vi "Autotest_Instr.vi"(8 "error in (no error)":errorcluster caption="entrée d'erreur (pas d'erreur)", 11 "Class Instrument (Default) en entrée":refnum<class "Class Instrument (Default).lvclass">) -> (0 "error out":errorcluster caption="sortie d'erreur", 3 "Class Instrument (Default) en sortie":refnum<class "Class Instrument (Default).lvclass">)   [LabVIEW 2020, in "Library Instrument & Equipement.lvlib" / "Library Instruments.lvlib" / "Class Instrument (Default).lvclass"]
uses:
  Class Instrument (Default).lvclass
  Class Instrument (Default).lvclass/Class Instrument (Default).ctl
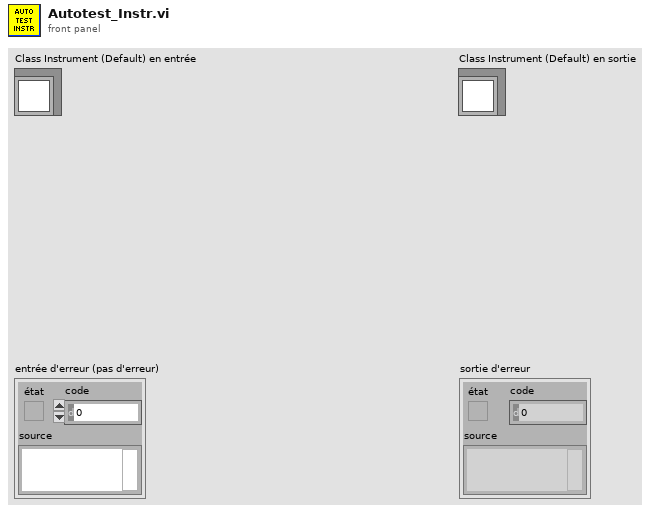
[diagram p1: front panel]
types:
  T1 = typedef "Semaphore RefNum" = refnum<k1>
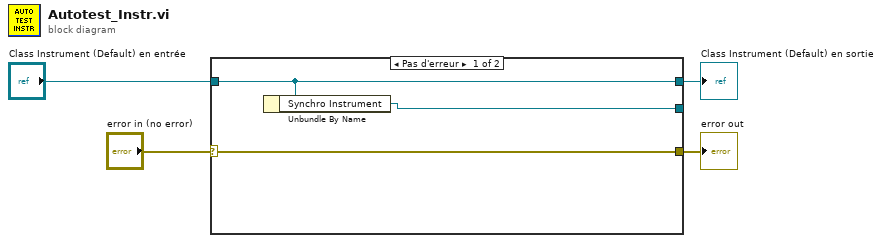
[diagram p0: block diagram]
diagram:
  n1 = case shown="Pas d'erreur" "error in (no error)" {
    selector: "error in (no error)" -> [w7 w9]
    tunnel: [w7 w9] -> w3
    tunnel: [w6 w8] -> w1
    tunnel: "Class Instrument (Default) en entrée" -> [w6 w8]
    tunnel: [w5 _] -> _
    frame No Error {
      n2 = Unbundle By Name(w6) -> ("Synchro Instrument"=w5:T1)
    }
    frame Error {
    }
  }
  "error out" <- w3
  "Class Instrument (Default) en sortie" <- w1
